vi "Init Events.vi"(8 "error in (no error)":errorcluster, 11 "DeviceArrayPanel in":refnum<class "DeviceArrayPanel.lvclass">) -> (0 "error out":errorcluster, 3 "DeviceArrayPanel out":refnum<class "DeviceArrayPanel.lvclass">)   [LabVIEW 2020, in "PicoG-App.lvlib" / "DeviceArrayPanel.lvclass"]
uses:
  DeviceArrayPanel.lvclass
  DeviceArrayPanel.lvclass/DeviceArrayPanel.ctl
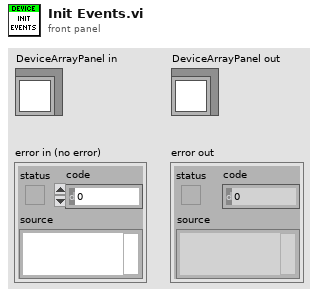
[diagram p1: front panel]
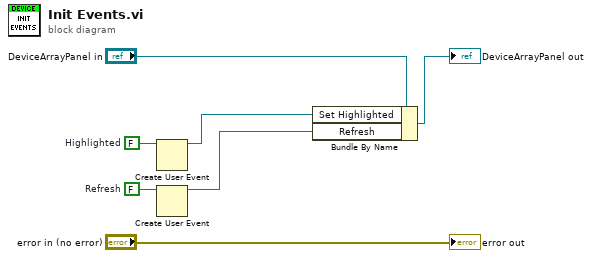
[diagram p0: block diagram]
diagram:
  w2 = FALSE  # Refresh
  w4 = FALSE  # Highlighted
  n1 = Create User Event(user event datatype=w4) -> (user event=w3:refnum<user-event>)  [unwired: 1 in, 1 out]
  n2 = Create User Event(user event datatype=w2) -> (user event=w1:refnum<user-event>)  [unwired: 1 in, 1 out]
  n3 = Bundle By Name(cluster="DeviceArrayPanel in", "Set Highlighted"=w3, "Refresh"=w1) -> (→"DeviceArrayPanel out":refnum<class "DeviceArrayPanel.lvclass">)
  "error out" <- "error in (no error)"
